vi "FixMgiMonitoredActor.vi"() -> ()   [LabVIEW 2020]
uses:
  <vilib>/Utility/EditLVLibs/Edit LVLibs.lvlib
  <vilib>/Utility/EditLVProj/Edit LVProj.lvlib
panel:
  out "Array":string[](array[string])
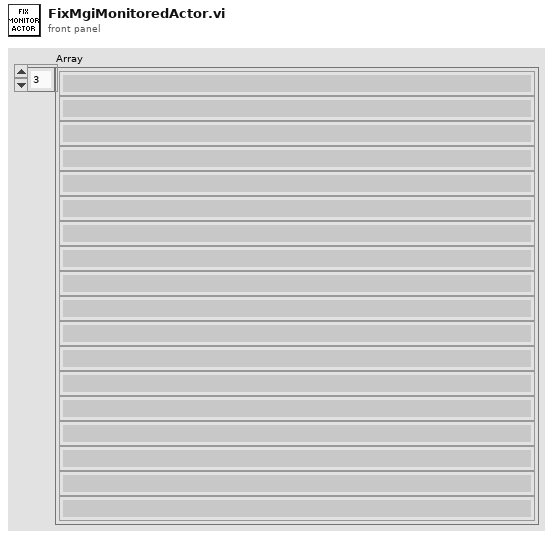
[diagram p1: front panel]
types:
  T1 = enum32{"Invalid", "Standard", "Closed", "Hidden", "Minimized", "Maximized"}
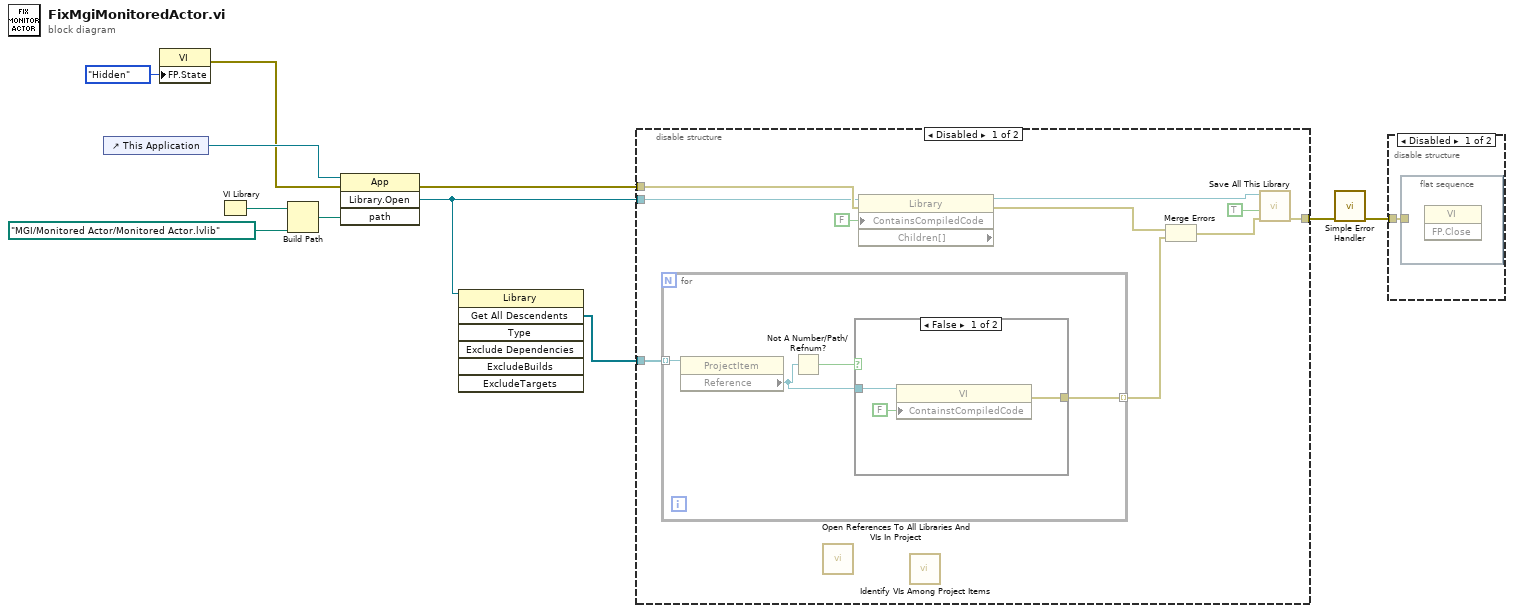
[diagram p0: block diagram]
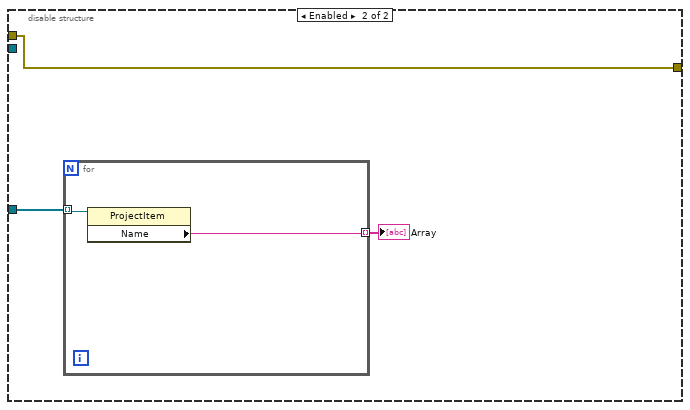
[diagram p4: hidden frame]
diagram:
  n1 = control-ref of="This Application"() -> (w8:refnum<vi>)
  n2 = property class="VI"("FP.State"=T1."Hidden" ("Front Panel Window:State")) -> (error out=w1:errorcluster)  [unwired: 2 in, 1 out]
  n3 = VI Library() -> (path=w5:path)
  n4 = Build Path(base path=w5, name or relative path=path "MGI/Monitored Actor/Monitored Actor.lvlib") -> (appended path=w7:path)
  n5 = invoke class="App" method="Library.Open"(reference=w8, error in=w1, "path"=w7) -> (error out=w10:errorcluster, "Open Library"=w4:refnum<vi>)  [unwired: 1 in, 2 out]
  n6 = invoke class="Library" method="Get All Descendents"(reference=w4) -> ("All Descendents"=w3:refnum<vi>[])  [unwired: 6 in, 6 out]
  n7 = disable-structure shown="Disabled" {
    disable-tunnel: w10 -> [w21 w31]
    disable-tunnel: [w20 w31] -> w9
    disable-tunnel: w4 -> [w13 _]
    disable-tunnel: w3 -> [w12 w30]
    frame Disabled {
      n8 = for {
        tunnel: [w25] -> w14 mode=indexing
        tunnel: w12 -> [w22] mode=indexing
        n9 = property class="ProjectItem"(reference=w22) -> ("Reference"=w23:refnum<vi>)  [unwired: 1 in, 2 out]
        n10 = Not A Number/Path/Refnum?(number/path/refnum=w23) -> (NaN/Path/Refnum?=w24:bool)
        n11 = case shown="False" w24 {
          tunnel: w23 -> [w26 _]
          tunnel: [w28 _] -> w25
          frame False {
            n12 = property class="VI"(reference=w26, "ContainstCompiledCode"=FALSE ("Contains Compiled Code")) -> (error out=w28:errorcluster)  [unwired: 1 in, 1 out]
          }
          frame True {
          }
        }
      }
      n13 = call <vilib>:"Open References To All Libraries And VIs In Project.vi"() -> ()  [unwired: 9 in, 3 out]
      n14 = property class="Library" props=["ContainsCompiledCode", "Children[]"](reference=w13, error in=w21, "ContainsCompiledCode"=FALSE ("Contains Compiled Code")) -> (reference out=w16:refnum<vi>, error out=w19:errorcluster)  [unwired: 1 out]
      n15 = call <vilib>:"Identify VIs Among Project Items.vi"() -> ()  [unwired: 10 in, 2 out]
      n16 = Merge Errors(w19, w14) -> (w18:errorcluster)
      n17 = call <vilib>:"Save All This Library.vi"("error in (no error)"=w18, "Save Only Modified VIs and Libraries? (F)"=TRUE, "Library in"=w16) -> ("error out"=w20:errorcluster)  [unwired: 7 in, 1 out]
    }
    frame Enabled {
      n18 = for {
        tunnel: w30 -> [w33] mode=indexing
        tunnel: [w32] -> w29 mode=indexing
        n19 = property class="ProjectItem"(reference=w33) -> ("Name"=w32:string)  [unwired: 1 in, 2 out]
      }
      "Array" <- w29
    }
  }
  n20 = call <vilib>:"Simple Error Handler.vi"("error in (no error)"=w9) -> ("error out"=w11:errorcluster)  [unwired: 4 in, 4 out]
  n21 = disable-structure shown="Disabled" {
    disable-tunnel: w11 -> [w34 _]
    frame Disabled {
      n22 = flat-sequence {
        tunnel: w34 -> [_]
        frame #0 {
          n23 = invoke class="VI" method="FP.Close"() -> ()  [unwired: 3 in, 3 out]
        }
      }
    }
    frame Enabled {
    }
  }
